vi "URUCHOMIENIE GEN 100kHz.vi"() -> ()   [LabVIEW 2013]
uses:
  <vilib>/DAQmx/create/channels.llb/DAQmx Create Channel (CO-Pulse Generation-Frequency).vi
  <resource>/objmgr/daqmx.rc
panel:
  out "dziala":bool
  in  "stop":bool
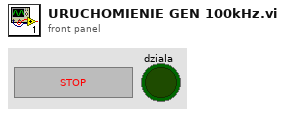
[diagram p1: front panel]
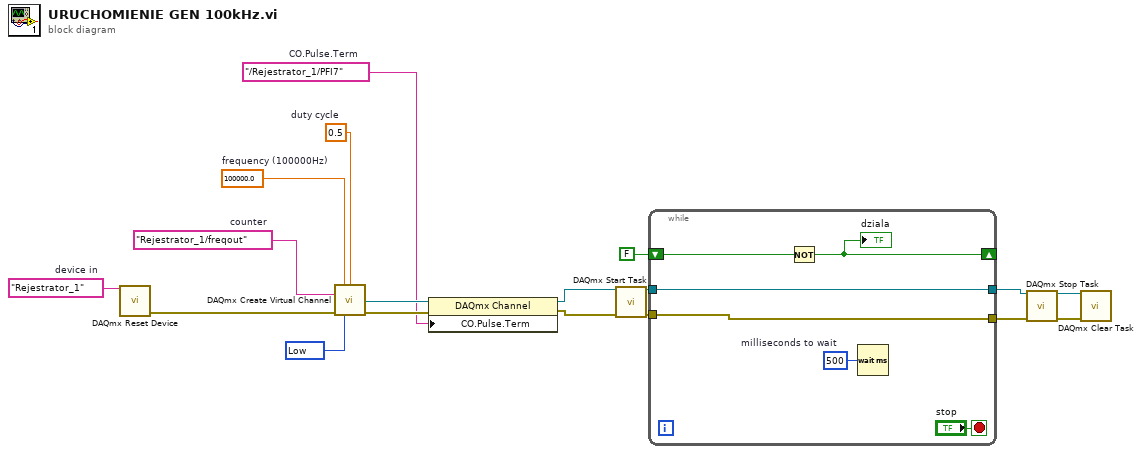
[diagram p0: block diagram]
diagram:
  w3 = tag "/Rejestrator_1/PFI7"  # CO.Pulse.Term
  w7 = 0.5  # duty cycle
  w8 = tag "Rejestrator_1"  # device in
  w15 = 100000.0  # frequency (100000Hz)
  w16 = tag "Rejestrator_1/freqout"  # counter
  w18 = 10214 items=["High"=10192, "Low"=10214] ("idle state")
  n1 = call <vilib>:"DAQmx Reset Device.vi"("device in"=w8) -> ("error out"=w17:errorcluster)  [unwired: 14 in]
  n2 = call-poly <vilib>:"DAQmx Create Virtual Channel.vi"("frequency"=w15, "duty cycle"=w7, "counter"=w16, "error in"=w17, "idle state"=w18) -> ("task out"=w4:refnum<k21>, "error out"=w6:errorcluster)  [unwired: 9 in]
  n3 = property class="DAQmx Channel"(reference=w4, error in=w6, "CO.Pulse.Term"=w3) -> (reference out=w2:refnum<k21>, error out=w5:errorcluster)
  n4 = call <vilib>:"DAQmx Start Task.vi"("task/channels in"=w2, "error in"=w5) -> ("task out"=w14:refnum<k21>, "error out"=w13:errorcluster)  [unwired: 12 in]
  n5 = while {
    tunnel: w14 -> [w22]
    tunnel: w13 -> [w23]
    tunnel: [w23] -> w10
    tunnel: [w22] -> w9
    shift-right: [w19] -> _
    shift-left: FALSE -> [w20]
    stop <- "stop" stop-if-true
    w21 = u32 500  # milliseconds to wait
    n6 = Not(x=w20) -> (.not. x?=w19:bool)
    "dziala" <- w19
    n7 = Wait (ms)(milliseconds to wait=w21) -> ()  [unwired: 1 out]
  }
  n8 = call <vilib>:"DAQmx Stop Task.vi"("task/channels in"=w9, "error in"=w10) -> ("task out"=w12:refnum<k21>, "error out"=w11:errorcluster)  [unwired: 12 in]
  n9 = call <vilib>:"DAQmx Clear Task.vi"("task in"=w12, "error in"=w11) -> ()  [unwired: 13 in, 1 out]
